vi "Read csv File.vi"(8 "error in (no error)":errorcluster caption="错误输入（无错误）", 11 "file path (dialog if empty)":path caption="文件路径 （空时为对话框）") -> (0 "error out":errorcluster caption="错误输出", 2 "all rows":string[][](array[string]) caption="所有行", 3 "new file path (Not A Path if cancelled)":path caption="新建文件路径（取消时为非法路径）")   [LabVIEW 2014]
panel:
  out "Address":T1(array[cluster])
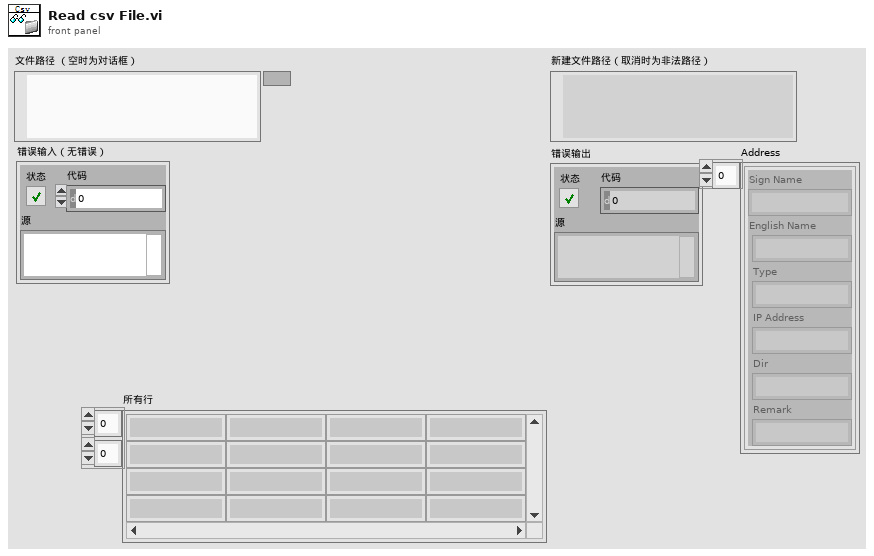
[diagram p1: front panel]
types:
  T1 = cluster{"Sign Name":string, "English Name":string, "Type":string, "IP Address":string, "Dir":string, "Remark":string}[]
  T2 = cluster{"Sign Name":string, "IP Address":string, "Type":string, "Target Address":string, "Dir":string, "Remark":string}[]
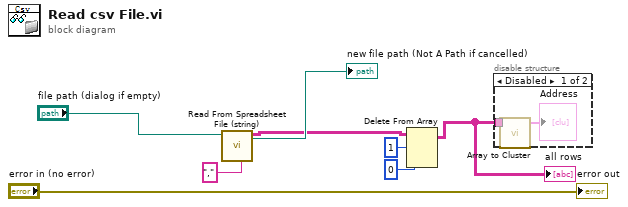
[diagram p0: block diagram]
diagram:
  n1 = call <vilib>:"Read From Spreadsheet File (string).vi"("delimiter (\\t)"="," ("delimiter (\\t)"), "file path (dialog if empty)"="file path (dialog if empty)") -> ("all rows"=w2:string[][], "new file path (Not A Path if cancelled)"=→"new file path (Not A Path if cancelled)":path)  [unwired: 5 in, 3 out]
  n2 = Delete From Array(array=w2, length=1, index (row)=0) -> (array with subset deleted=w1:string[][])  [unwired: 1 in, 1 out]
  "all rows" <- w1
  n3 = disable-structure shown="Disabled" {
    disable-tunnel: w1 -> [w9 _]
    frame Disabled {
      n4 = call "Array to Cluster.vi"("2D Array"=w9) -> ("Address"=→"Address":T2)  [unwired: 4 in]
    }
    frame Enabled {
    }
  }
  "error out" <- "error in (no error)"
